vi "Front Camera Circle detect.vi"() -> ()   [LabVIEW 2014]
uses:
  <vilib>/vision/Shape Detection.llb/ShapeDetectionMatchOptions.ctl
  <vilib>/vision/Pattern Matching.llb/IMAQ Match Range Setting.ctl
  <vilib>/vision/Pattern Matching.llb/IMAQ Curve Parameters.ctl
  Global.vi
  <vilib>/vision/NI_Vision_Development_Module.lvlib
panel:
  in  "Circle Index":i32
  out "Score":dbl
  out "Number of Matches Returned":i32
  in  "Curve Parameters":T1={"Extraction Mode"=0, "Edge Threshold"=150, "Edge Filter Size"=1, "Min Length"=25, "Row Search Step Size"=15, "Col Search Step Size"=15, "Max Endpoint Gap"=10, "Closed"=TRUE, "Subpixel"=FALSE} {"Extraction Mode" items=["Normal", "Uniform Regions"]; "Edge Filter Size" items=["Fine", "Normal", "Contour Tracing"]; "Max Endpoint Gap" min=0; "Col Search Step Size" min=1 max=255 step=1; "Row Search Step Size" min=1 max=255 step=1; "Min Length" min=0; "Edge Threshold" min=1 max=350 step=1}
  out "error out":errorcluster
  in  "Minimum match score":dbl=900.0
  in  "Match Options":T2={"Rotation"=FALSE, "Scale"=FALSE, "Occlusion"=TRUE, "Range Settings"=[{"Match Constraints"=0, "Min"=0.0, "Max"=0.0}, {"Match Constraints"=1, "Min"=0.0, "Max"=0.0}, {"Match Constraints"=2, "Min"=0.0, "Max"=25.0}]} {"Range Settings"."Max" format="%.2f"; "Range Settings"."Min" format="%.2f"; "Range Settings"."Match Constraints" items=["Rotation Angle (degrees)", "Scale Factor (%)", "Occlusion (%)"]}
  in  "Circle Descriptor":cluster{"Min Radius":dbl, "Max Radius":dbl}={"Min Radius"=20.0, "Max Radius"=400.0}
  out "Image":T4(plugin-control)
  in  "stop video":bool
  in  "milliseconds to wait":u32
  out "Read Video":errorcluster
  out "x-y":u32=19
  # "Range"
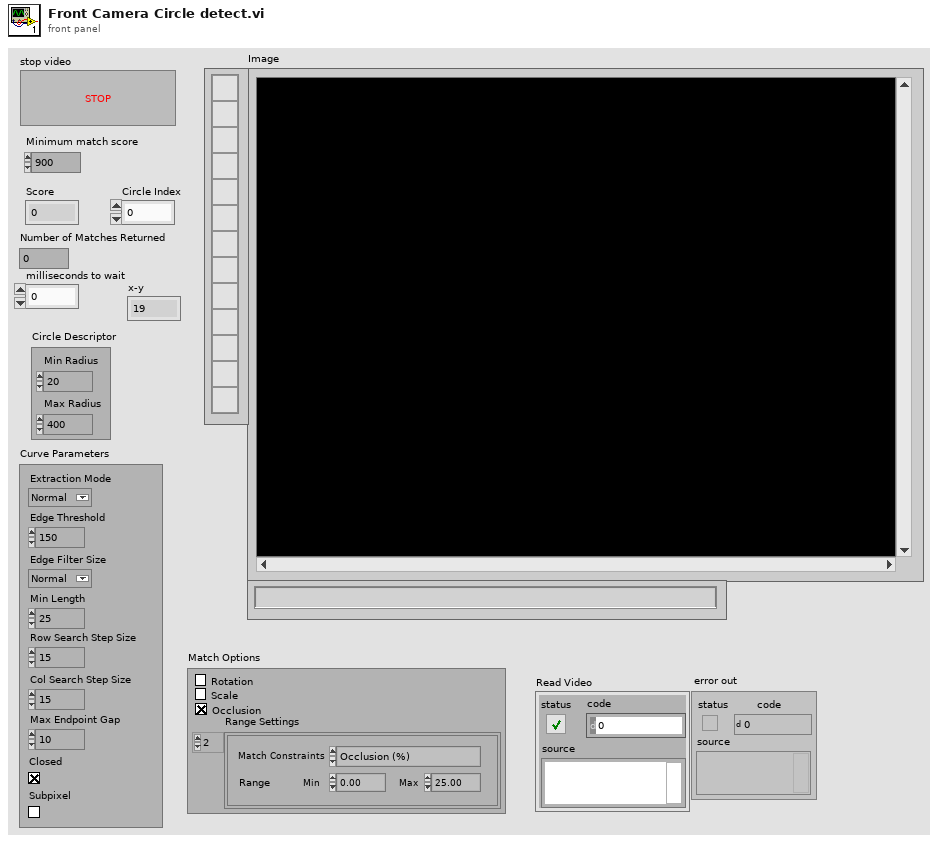
[diagram p1: front panel]
types:
  T1 = typedef "IMAQ Curve Parameters.ctl" = cluster{"Extraction Mode":u32, "Edge Threshold":i32, "Edge Filter Size":u32, "Min Length":i32, "Row Search Step Size":i32, "Col Search Step Size":i32, "Max Endpoint Gap":i32, "Closed":bool, "Subpixel":bool}
  T2 = typedef "ShapeDetectionMatchOptions.ctl" = cluster{"Rotation":bool, "Scale":bool, "Occlusion":bool, "Range Settings":T3[]}
  T3 = typedef "IMAQ Match Range Setting.ctl" = cluster{"Match Constraints":u32, "Min":dbl, "Max":dbl}
  T4 = typedef "IMAQ Image.ctl" = refnum<image>
  T5 = typedef "Image Type" = u32
  T6 = cluster{"Position":cluster{"X":sgl, "Y":sgl}, "Radius":dbl, "Score":dbl}[]
  T7 = cluster{"Position":cluster{"X":sgl, "Y":sgl}, "Radius":dbl, "Score":dbl}
  T8 = cluster{"Left":i32, "Top":i32, "Right":i32, "Bottom":i32}
  T9 = typedef "Control cluster.ctl" = cluster{"Roll":sgl, "Pitch":sgl, "Vertical Speed":sgl, "Yaw Speed":sgl}
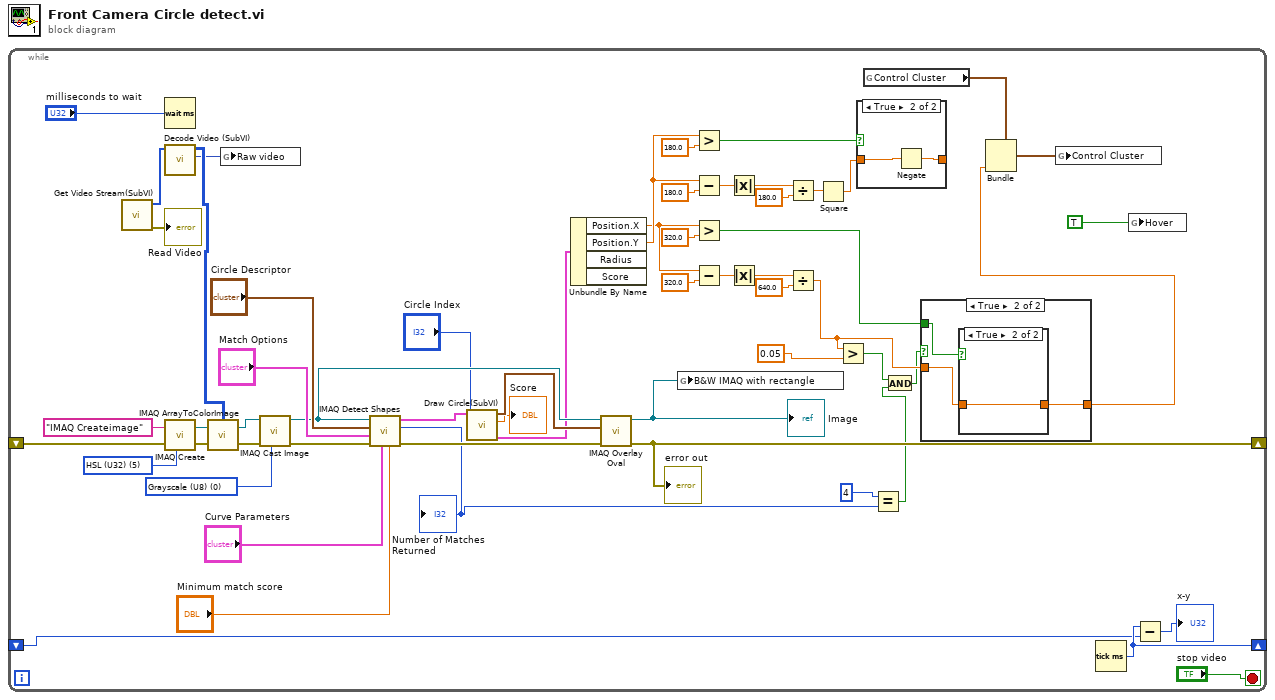
[diagram p0: block diagram]
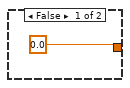
[diagram p2: hidden frame]
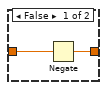
[diagram p3: hidden frame]
diagram:
  n1 = while {
    shift-right: [w49] -> _
    shift-left: _ -> [w48]
    shift-right: [w34] -> _
    shift-left: _ -> [w45]
    stop <- "stop video" stop-if-true
    w42 = T5 0 items=["Grayscale (U8)", "Grayscale (I16)", "Grayscale (SGL)", "Complex (CSG)", "RGB (U32)", "HSL (U32)", "RGB (U64)", "Grayscale (U16)"] ("Image Type")
    w55 = T5 5 items=["Grayscale (U8)", "Grayscale (I16)", "Grayscale (SGL)", "Complex (CSG)", "RGB (U32)", "HSL (U32)", "RGB (U64)", "Grayscale (U16)"] ("Image Type")
    n2 = call "Get Video Stream(SubVI).vi"() -> ("error out"=→"Read Video":errorcluster, "ImgData"=w56:u8[])  [unwired: 10 in]
    n3 = Wait (ms)(milliseconds to wait="milliseconds to wait") -> ()  [unwired: 1 out]
    n4 = call "Decode Video (SubVI).vi"("ImgData"=w56) -> ("new picture"=w46:picture, "Array"=w52:u32[][])  [unwired: 9 in]
    n5 = call "IMAQ Create"("Image Name"="IMAQ Createimage", "Image Type"=w55, "error in (no error)"=w45) -> ("New Image"=w51:T4, "error out"=w50:errorcluster)  [unwired: 2 in]
    n6 = call "IMAQ ArrayToColorImage"("Image Pixels (U32)"=w52, "Image"=w51, "error in (no error)"=w50) -> ("Image Out"=w43:T4, "error out"=w44:errorcluster)  [unwired: 2 in]
    n7 = global write "Global.vi" "Raw video"(w46) -> ()
    n8 = call "IMAQ Cast Image"("Image Type"=w42, "error in (no error)"=w44, "Image Src"=w43) -> ("error out"=w39:errorcluster, "Image Dst Out"=w37:T4)  [unwired: 7 in]
    n9 = call-poly "IMAQ Detect Shapes"("Minimum match score"="Minimum match score", "Curve Parameters"="Curve Parameters", "error in (no error)"=w39, "Match Options"="Match Options", "Circle Descriptor"="Circle Descriptor", "Image"=w37) -> ("error out"=w36:errorcluster, "Number of Matches Returned"=w6:i32, "Circles"=w32:T6)  [unwired: 3 in]
    "Number of Matches Returned" <- w6
    n10 = call "Draw Circle(SubVI).vi"("Circle Index"="Circle Index", "Circles"=w32) -> ("element"=w30:T7, "Score"=→"Score":dbl, "Bounding Rectangle out"=w35:T8)  [unwired: 7 in]
    n11 = Unbundle By Name(w30) -> ("Position.X"=w15:sgl, "Position.Y"=w20:sgl)  [unwired: 2 out]
    n12 = call "IMAQ Overlay Oval"("error in (no error)"=w36, "Bounding Rectangle"=w35, "Image"=w37) -> ("error out"=w34:errorcluster, "Image Out"=w28:T4)  [unwired: 7 in]
    "Image" <- w28
    "error out" <- w34
    n13 = global write "Global.vi" "B&W IMAQ with rectangle"(w28) -> ()
    n14 = Greater?(x=w20, y=180.0) -> (0:w26:bool)
    n15 = Subtract(x=w20, y=180.0) -> (x-y=w23:dbl)
    n16 = Greater?(x=w15, y=320.0) -> (0:w10:bool)
    n17 = Subtract(x=w15, y=320.0) -> (x-y=w18:dbl)
    n18 = Absolute Value(x=w23) -> (abs(x)=w22:dbl)
    n19 = Absolute Value(x=w18) -> (abs(x)=w17:dbl)
    n20 = Divide(x=w22, y=180.0) -> (x/y=w13:dbl)
    n21 = Divide(x=w17, y=640.0) -> (x/y=w8:dbl)
    n22 = Square(x=w13) -> (x^2=w14:dbl)
    n23 = Greater?(x=w8, y=0.05) -> (0:w2:bool)
    n24 = case shown="True" w26 {
      tunnel: w14 -> [w66 w68]
      tunnel: [w66 w67] -> _
      frame False {
      }
      frame True {
        n25 = Negate(x=w68) -> (-x=w67:dbl)
      }
    }
    n26 = global read "Global.vi" "Control Cluster"() -> (w12:T9)
    n27 = Equal?(x=4, y=w6) -> (x = y?=w3:bool)
    n28 = And(x=w2, y=w3) -> (x .and. y?=w4:bool)
    n29 = case shown="True" w4 {
      tunnel: w10 -> [_ w62]
      tunnel: [0.0 w61] -> w9
      tunnel: w8 -> [_ w60]
      frame False {
      }
      frame True {
        n30 = case shown="True" w62 {
          tunnel: w60 -> [w64 w65]
          tunnel: [w63 w65] -> w61
          frame False {
            n31 = Negate(x=w64) -> (-x=w63:dbl)
          }
          frame True {
          }
        }
      }
    }
    n32 = Bundle(cluster=w12, "Yaw Speed"=w9) -> (w29:T9)  [unwired: 3 in]
    n33 = global write "Global.vi" "Control Cluster"(w29) -> ()
    n34 = Tick Count (ms)() -> (millisecond timer value=w49:u32)
    n35 = global write "Global.vi" "Hover"(TRUE) -> ()
    n36 = Subtract(x=w49, y=w48) -> (x-y=→"x-y":u32)
  }
